vi "fiber_spiral_parameters_to_FPGA_cycle_parameters.vi"(8 "error in (no error)":errorcluster, 10 "Fiber spiral parameters":T3={"Fiber Frequency"=2200, "Imaging Periods"=100, "Settling Periods"=50, "Resting Periods"=30, "Amplitude X"=0.5, "Amplitude Y"=0.5, "Phase difference"=90.0, "Initial Amplitude X"=0.0, "Initial Amplitude Y"=0.0} {"Initial Amplitude Y" min=0.0 max=3.0 step=0.1; "Initial Amplitude X" min=0.0 max=3.0 step=0.1; "Phase difference" min=0.0 max=360.0 step=5.0; "Amplitude Y" min=0.0 max=3.0 step=0.1; "Amplitude X" min=0.0 max=3.0 step=0.1}, 11 "FPGAWrapperRK120511Fiber_Spiral in":refnum<class "FPGAWrapperRK110512Fiber_Spiral.lvclass">) -> (0 "error out":errorcluster, 2 "FPGA Cycle Parameters XY":T1={"FPGA Cycle Parameters X"={"Imaging cycles"=285714, "Settling cycles"=71429, "Resting cycles"=42857, "Phase advance per cycle"=0.0001399517059326172, "Imaging Multiplier advance per cycle"=0.00286865234375, "Settling Multiplier advance per cycle"=-0.0057373046875, "Imaging Initial Multiplier"=0.0, "Initial Phase"=0.0}, "FPGA Cycle Parameters Y"={"Imaging cycles"=285714, "Settling cycles"=71429, "Resting cycles"=42857, "Phase advance per cycle"=0.0001399517059326172, "Imaging Multiplier advance per cycle"=0.00286865234375, "Settling Multiplier advance per cycle"=-0.0057373046875, "Imaging Initial Multiplier"=0.0, "Initial Phase"=0.0}}, 3 "FPGAWrapperRK120511Fiber_Spiral out":refnum<class "FPGAWrapperRK110512Fiber_Spiral.lvclass">)   [LabVIEW 2010, in "FPGAWrapperRK110512Fiber_Spiral.lvclass"]
uses:
  FPGAWrapperRK110512Fiber_Spiral.lvclass
  fiber_spiral_parameters.ctl
  FPGA_Typedefs/FPGA Cycle Parameters XY.ctl
  FPGA_Typedefs/FPGA Cycle Parameters.ctl
  FPGAWrapperRK110512Fiber_Spiral.lvclass/FPGAWrapperRK110512Fiber_Spiral.ctl
panel:
  # "[Hz]"
  # "[V]"
  # "[V]"
  # "[deg]"
  # "[V]"
  # "[V]"
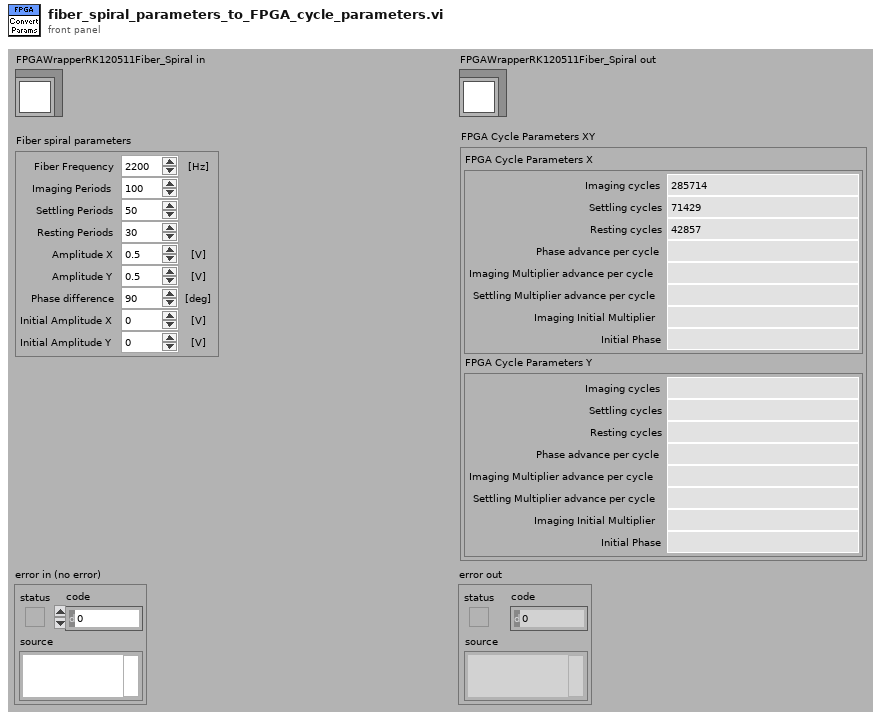
[diagram p1: front panel]
types:
  T1 = typedef "FPGA Cycle Parameters XY.ctl" = cluster{"FPGA Cycle Parameters X":T2, "FPGA Cycle Parameters Y":T2}
  T2 = typedef "FPGA Cycle Parameters.ctl" = cluster{"Imaging cycles":i32, "Settling cycles":i32, "Resting cycles":i32, "Phase advance per cycle":fxp<+,32,0>, "Imaging Multiplier advance per cycle":fxp<+/-,32,0>, "Settling Multiplier advance per cycle":fxp<+/-,32,0>, "Imaging Initial Multiplier":fxp<+/-,43,12>, "Initial Phase":fxp<+,32,1>}
  T3 = typedef "FPGAWrapperRK110512Fiber_Spiral.lvclass/fiber_spiral_parameters.ctl" = cluster{"Fiber Frequency":u16, "Imaging Periods":u16, "Settling Periods":u16, "Resting Periods":u16, "Amplitude X":dbl, "Amplitude Y":dbl, "Phase difference":dbl, "Initial Amplitude X":dbl, "Initial Amplitude Y":dbl}
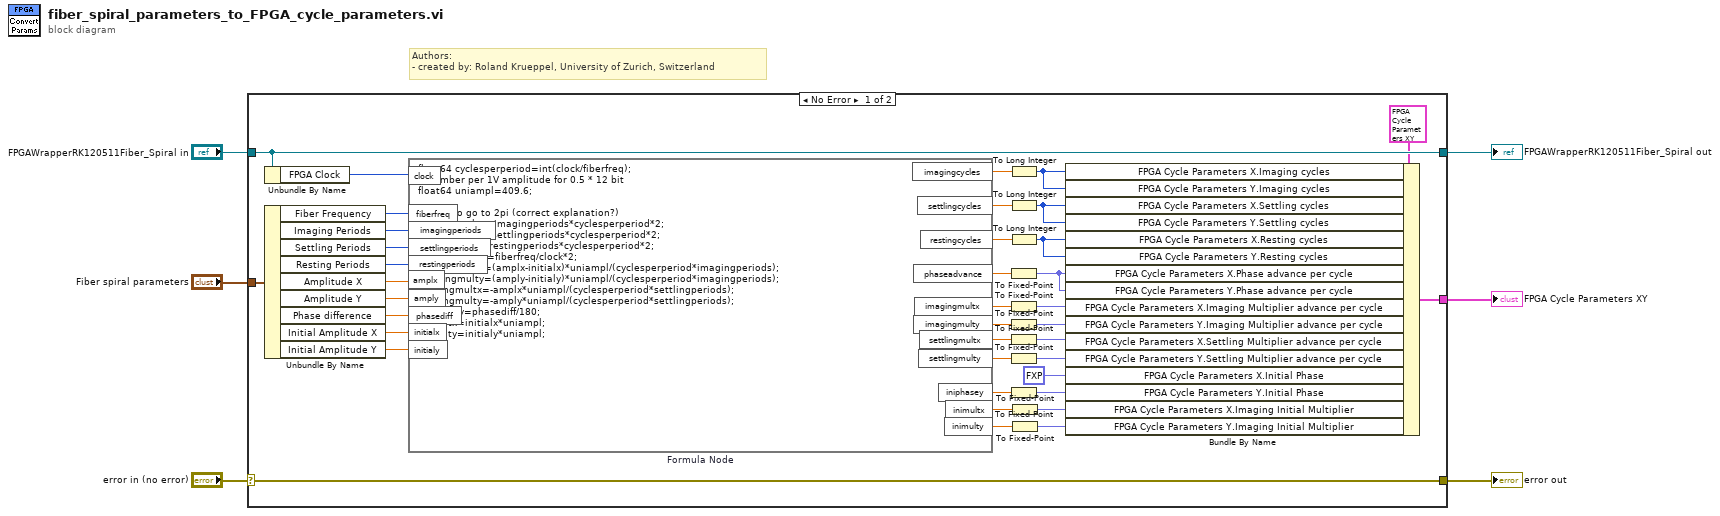
[diagram p0: block diagram]
diagram:
  # "Authors: \n- created by: Roland Krueppel, University of Zurich, Switzerland"
  n1 = case shown="No Error" "error in (no error)" {
    selector: "error in (no error)" -> [w44 w46]
    tunnel: [w44 w46] -> w5
    tunnel: [w10 w45] -> w3
    tunnel: "FPGAWrapperRK120511Fiber_Spiral in" -> [w10 w45]
    tunnel: "Fiber spiral parameters" -> [w9 _]
    tunnel: [w7 _] -> w1
    frame No Error {
      n2 = Unbundle By Name(w10) -> ("FPGA Clock"=w34:u32)
      n3 = Unbundle By Name(w9) -> ("Fiber Frequency"=w43:u16, "Imaging Periods"=w42:u16, "Settling Periods"=w41:u16, "Resting Periods"=w40:u16, "Amplitude X"=w39:dbl, "Amplitude Y"=w38:dbl, "Phase difference"=w37:dbl, "Initial Amplitude X"=w36:dbl, "Initial Amplitude Y"=w35:dbl)
      n4 = formula code="float64 cyclesperperiod=int(clock/fiberfreq);\n// Number per 1V amplitude for 0.5 * 12 bit\nfloat64 uniampl=409.6;\n\n// have to go to 2pi (correct explanation?)\nimagingcycles=imagingperiods*cyclesperperiod*2;\nsettlingcycles=settlingperiods*cyclesperperiod*2;\nrestingcycles=restingperiods*cyclesperperiod*2;\nphaseadvance=fiberfreq/clock*2;\nimagingmultx=(amplx-initialx)*uniampl/(cyclesperperiod*imagingperiods);\nimagingmulty=(amply-initialy)*uniampl/(cyclesperperiod*imagingperiods);\nsettlingmultx=-amplx*uniampl/(cyclesperperiod*settlingperiods);\nsettlingmulty=-amply*uniampl/(cyclesperperiod*settlingperiods);\niniphasey=phasediff/180;\ninimultx=initialx*uniampl;\ninimulty=initialy*uniampl;"("fiberfreq"=w43, "imagingperiods"=w42, "settlingperiods"=w41, "restingperiods"=w40, "amplx"=w39, "amply"=w38, "phasediff"=w37, "initialx"=w36, "initialy"=w35, "clock"=w34) -> ("imagingcycles"=w21:dbl, "settlingcycles"=w20:dbl, "restingcycles"=w19:dbl, "phaseadvance"=w18:dbl, "imagingmultx"=w17:dbl, "imagingmulty"=w16:dbl, "iniphasey"=w13:dbl, "inimultx"=w12:dbl, "inimulty"=w11:dbl, "settlingmultx"=w15:dbl, "settlingmulty"=w14:dbl)
      n5 = To Long Integer(number=w21) -> (32bit integer=w28:i32)
      n6 = To Long Integer(number=w20) -> (32bit integer=w27:i32)
      n7 = To Long Integer(number=w19) -> (32bit integer=w26:i32)
      n8 = To Fixed-Point(number=w18) -> (fixed-point=w31:fxp<+,32,0>)  [unwired: 1 in]
      n9 = To Fixed-Point(number=w17) -> (fixed-point=w33:fxp<+/-,32,0>)  [unwired: 1 in]
      n10 = To Fixed-Point(number=w16) -> (fixed-point=w30:fxp<+/-,32,0>)  [unwired: 1 in]
      n11 = To Fixed-Point(number=w15) -> (fixed-point=w32:fxp<+/-,32,0>)  [unwired: 1 in]
      n12 = To Fixed-Point(number=w14) -> (fixed-point=w29:fxp<+/-,32,0>)  [unwired: 1 in]
      n13 = To Fixed-Point(number=w13) -> (fixed-point=w25:fxp<+,32,1>)  [unwired: 1 in]
      n14 = To Fixed-Point(number=w12) -> (fixed-point=w23:fxp<+/-,43,12>)  [unwired: 1 in]
      n15 = To Fixed-Point(number=w11) -> (fixed-point=w22:fxp<+/-,43,12>)  [unwired: 1 in]
      n16 = Bundle By Name(cluster=T1 {"FPGA Cycle Parameters X"={"Imaging cycles"=285714, "Settling cycles"=71429, "Resting cycles"=42857, "Phase advance per cycle"=0.0001399517059326172, "Imaging Multiplier advance per cycle"=0.00286865234375, "Settling Multiplier advance per cycle"=-0.0057373046875, "Imaging Initial Multiplier"=0.0, "Initial Phase"=0.0}, "FPGA Cycle Parameters Y"={"Imaging cycles"=285714, "Settling cycles"=71429, "Resting cycles"=42857, "Phase advance per cycle"=0.0001399517059326172, "Imaging Multiplier advance per cycle"=0.00286865234375, "Settling Multiplier advance per cycle"=-0.0057373046875, "Imaging Initial Multiplier"=0.0, "Initial Phase"=0.0}} ("FPGA Cycle Parameters XY"), "FPGA Cycle Parameters X.Imaging cycles"=w28, "FPGA Cycle Parameters Y.Imaging cycles"=w28, "FPGA Cycle Parameters X.Settling cycles"=w27, "FPGA Cycle Parameters Y.Settling cycles"=w27, "FPGA Cycle Parameters X.Resting cycles"=w26, "FPGA Cycle Parameters Y.Resting cycles"=w26, "FPGA Cycle Parameters X.Phase advance per cycle"=w31, "FPGA Cycle Parameters Y.Phase advance per cycle"=w31, "FPGA Cycle Parameters X.Imaging Multiplier advance per cycle"=w33, "FPGA Cycle Parameters Y.Imaging Multiplier advance per cycle"=w30, "FPGA Cycle Parameters X.Settling Multiplier advance per cycle"=w32, "FPGA Cycle Parameters Y.Settling Multiplier advance per cycle"=w29, "FPGA Cycle Parameters X.Initial Phase"=fxp<+,32,1> 0.0, "FPGA Cycle Parameters Y.Initial Phase"=w25, "FPGA Cycle Parameters X.Imaging Initial Multiplier"=w23, "FPGA Cycle Parameters Y.Imaging Initial Multiplier"=w22) -> (w7:T1)
    }
    frame Error {
    }
  }
  "error out" <- w5
  "FPGAWrapperRK120511Fiber_Spiral out" <- w3
  "FPGA Cycle Parameters XY" <- w1
